vi "Default Instrument Setup.vi"(8 "error in (no error)":errorcluster, 11 "VISA resource name":refnum<visa-resource-name>) -> (0 "error out":errorcluster, 3 "VISA resource name out":refnum<visa-resource-name>)   [LabVIEW 2024, in "Keithley DMM6500 DAQ6500 Series.lvlib"]
doc: "Sends a default command string to the instrument whenever a new VISA session is opened, or the instrument is reset. Use this VI as a subVI for the <b>Initialize</b> and <b>Reset</b> VIs. Altering this VI could cause these two VIs to operate incorrectly."
uses:
  Keithley DMM6500 DAQ6500 Series.lvlib
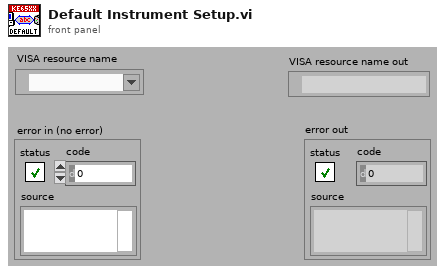
[diagram p1: front panel]
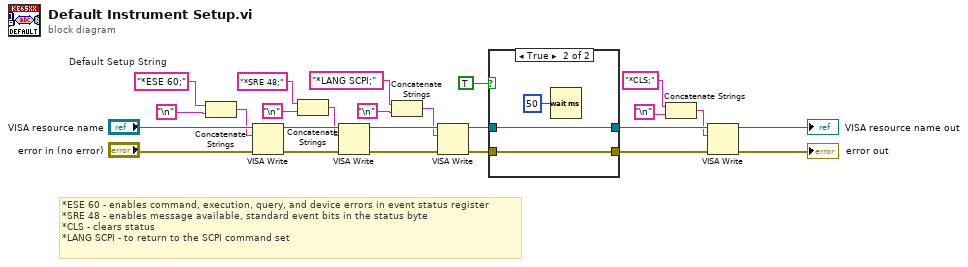
[diagram p0: block diagram]
diagram:
  w12 = "*ESE 60;"  # Default Setup String
  # "*ESE 60 - enables command, execution, query, and device errors in event status register\n*SRE 48 - enables message available, standard event bits in the status byte\n*CLS - clears status\n*LANG SCPI - to return to the SCPI command set"
  n1 = Concatenate Strings(w12, "\n") -> (w14:string)
  n2 = VISA Write(VISA resource name="VISA resource name", write buffer=w14, error in (no error)="error in (no error)") -> (VISA resource name out=w23:refnum<visa-resource-name>, error out=w22:errorcluster)  [unwired: 1 out]
  n3 = Concatenate Strings("*SRE 48;" ("write buffer"), "\n") -> (w19:string)
  n4 = VISA Write(VISA resource name=w23, write buffer=w19, error in (no error)=w22) -> (VISA resource name out=w21:refnum<visa-resource-name>, error out=w20:errorcluster)  [unwired: 1 out]
  n5 = Concatenate Strings("*LANG SCPI;" ("write buffer"), "\n") -> (w15:string)
  n6 = VISA Write(VISA resource name=w21, write buffer=w15, error in (no error)=w20) -> (VISA resource name out=w10:refnum<visa-resource-name>, error out=w9:errorcluster)  [unwired: 1 out]
  n7 = case shown="True" TRUE {
    tunnel: w10 -> [w27 w29]
    tunnel: w9 -> [w26 w28]
    tunnel: [w27 w29] -> w8
    tunnel: [w26 w28] -> w7
    frame False {
    }
    frame True {
      n8 = Wait (ms)(milliseconds to wait=u32 50) -> ()  [unwired: 1 out]
    }
  }
  n9 = Concatenate Strings("*CLS;" ("write buffer"), "\n") -> (w4:string)
  n10 = VISA Write(VISA resource name=w8, write buffer=w4, error in (no error)=w7) -> (VISA resource name out=→"VISA resource name out":refnum<visa-resource-name>, error out=→"error out":errorcluster)  [unwired: 1 out]
